vi "Synchronize Setting.vi"(8 "error in (no error)":errorcluster, 11 "Node Actor in":refnum<class "Node Actor.lvclass">) -> (0 "error out":errorcluster, 3 "Node Actor out":refnum<class "Node Actor.lvclass">)   [LabVIEW 2024, in "Node Actor.lvclass"]
uses:
  Node Actor.lvclass
  Node Actor.lvclass/Node Actor.ctl
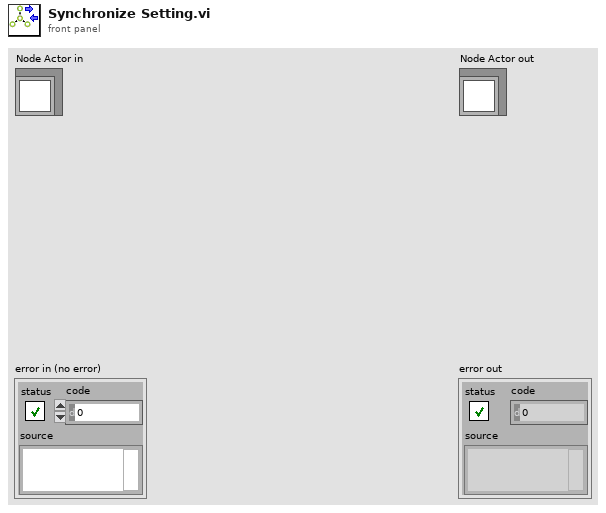
[diagram p1: front panel]
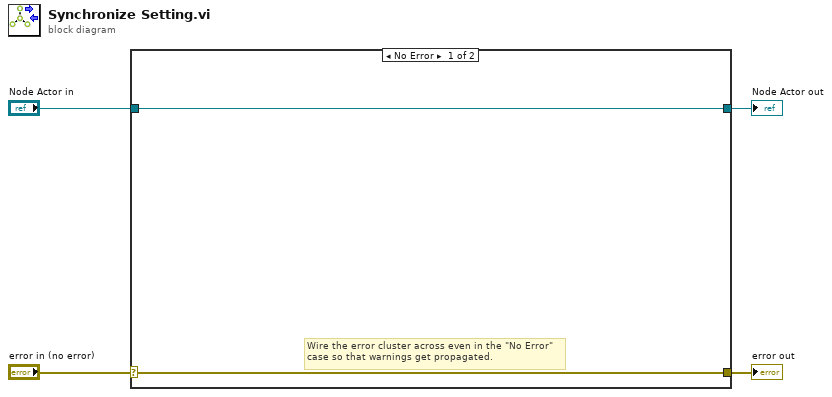
[diagram p0: block diagram]
diagram:
  n1 = case shown="No Error" "error in (no error)" {
    selector: "error in (no error)" -> [w5 w8]
    tunnel: [w5 w8] -> w3
    tunnel: [w6 w7] -> w1
    tunnel: "Node Actor in" -> [w6 w7]
    frame No Error {
      # "Wire the error cluster across even in the \"No Error\"\ncase so that warnings get propagated."
    }
    frame Error {
    }
  }
  "error out" <- w3
  "Node Actor out" <- w1
